vi "Read Report Display.vi"(8 "error in (no error)":errorcluster, 11 "Reports in":refnum<class "Results.lvclass">) -> (0 "error out":errorcluster, 2 "Report Display":refnum<vi>, 3 "Reports out":refnum<class "Results.lvclass">)   [LabVIEW 2016, in "Result Actor.lvlib" / "Results.lvclass"]
uses:
  <userlib>/Common Components/Results/Results.lvclass
  <userlib>/Common Components/Results/Results.lvclass/Results.ctl
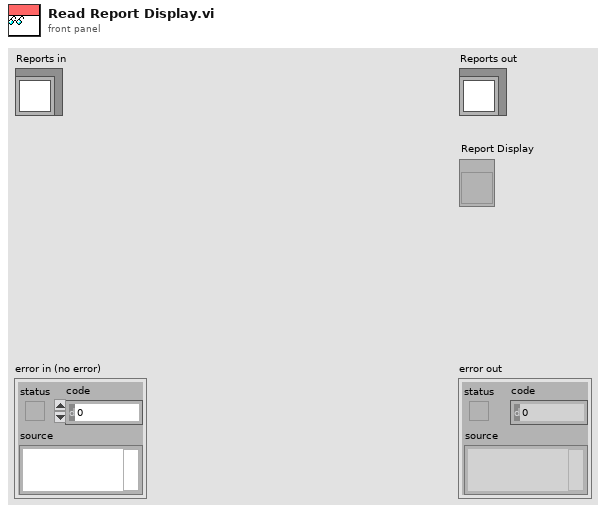
[diagram p1: front panel]
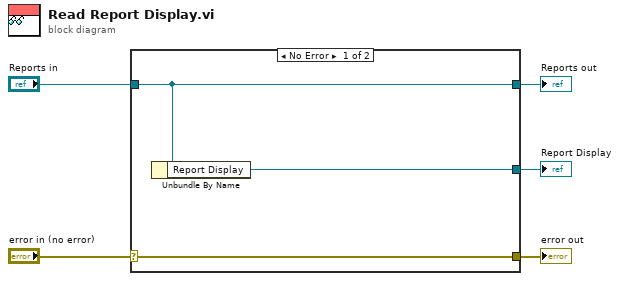
[diagram p0: block diagram]
diagram:
  n1 = case shown="No Error" "error in (no error)" {
    selector: "error in (no error)" -> [w8 w9]
    tunnel: [w8 w9] -> w4
    tunnel: [w7 w10] -> w2
    tunnel: "Reports in" -> [w7 w10]
    tunnel: [w6 _] -> w1
    frame No Error {
      n2 = Unbundle By Name(w7) -> ("Report Display"=w6:refnum<vi>)
    }
    frame Error {
    }
  }
  "error out" <- w4
  "Reports out" <- w2
  "Report Display" <- w1
